vi "Check Validity of Selection.vi"(8 "error in (no error)":errorcluster, 10 "valid":bool, 11 "Message Enqueuer in":refnum<class "Message Enqueuer.lvclass">) -> (0 "error out":errorcluster, 3 "Message Enqueuer out":refnum<class "Message Enqueuer.lvclass">)   [LabVIEW 2016, in "Controller UI.lvlib" / "Check Validity of Selection.lvclass"]
uses:
  <userlib>/Common Components/Controller UI/Messages/Check Run Button/Check Validity of Selection.lvclass
  <vilib>/ActorFramework/Message Enqueuer/Message Enqueuer.lvclass
  C:/Program Files (x86)/National Instruments/LabVIEW 2016/vi.lib/ActorFramework/Message/Message.lvclass
  <userlib>/Common Components/Controller UI/Messages/Check Run Button/Check Validity of Selection.lvclass/Check Validity of Selection.ctl
  <vilib>/ActorFramework/Message Enqueuer/Message Enqueuer.lvclass/Message Enqueuer.ctl
  <vilib>/ActorFramework/Message Priority Queue/Priority Enqueue.vi
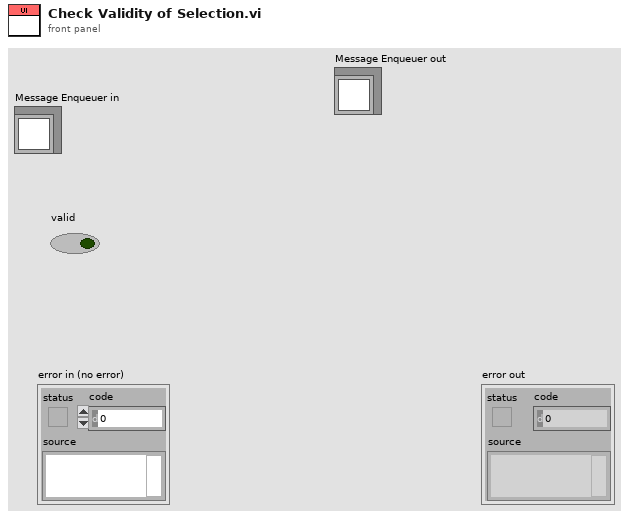
[diagram p1: front panel]
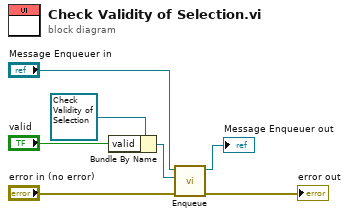
[diagram p0: block diagram]
diagram:
  n1 = Bundle By Name(cluster=refnum<class "Check Validity of Selection.lvclass"> refnum ("Check Validity of Selection.lvclass"), "valid"="valid") -> (w2:refnum<class "Check Validity of Selection.lvclass">)
  n2 = call <vilib>:"Enqueue.vi"("error in (no error)"="error in (no error)", "Message"=w2, "Message Enqueuer in"="Message Enqueuer in") -> ("error out"=→"error out":errorcluster, "Message Enqueuer out"=→"Message Enqueuer out":refnum<class "Message Enqueuer.lvclass">)  [unwired: 7 in]
